vi "DLL-based calc.vi"() -> ()   [LabVIEW 2018]
uses:
  D:/Users_Data/Dmitriy_T/Documents/Tracker/TestVI's/Calculus2/Calculus.dll
  Calculus.dll
  <userlib>/_OpenG.lib/numeric/numeric.llb/Random Number Within Range - DBL__ogtk.vi
  <vilib>/Analysis/NI_AALBase.lvlib
panel:
  out "size(s)":i32
  out "Image Display":T1(plugin-control)
  in  "Y":i32=250
  in  "X":i32=300
  in  "Image":bool
  out "variance, us":dbl format="%0.2f"
  out "standard deviation, us":dbl format="%0.2f"
  out "mean per cycle, us":dbl format="%0.2f"
  in  "N tests":i32=10000
  out "Randoms":T2(graph)
  out "error out":errorcluster
  in  "Exit button":bool
  in  "Subtract":bool
  in  "Add":bool
  out "Result":i32
  in  "B":i32
  in  "A":i32
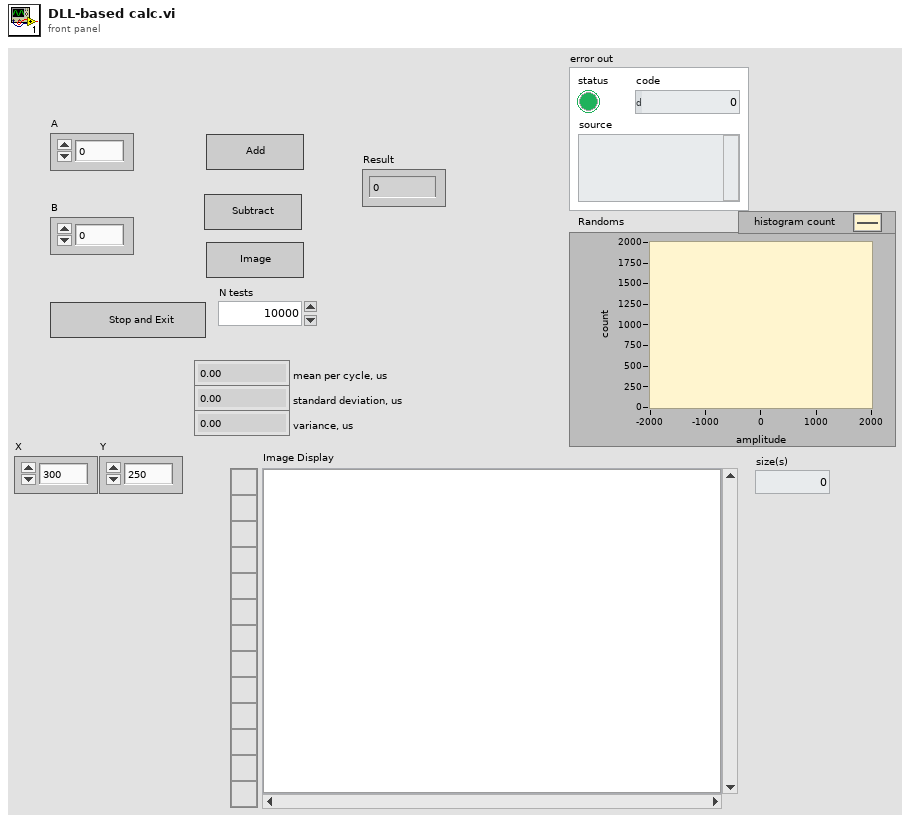
[diagram p1: front panel]
types:
  T1 = typedef "IMAQ Image.ctl" = refnum<image>
  T2 = cluster{"X Values":dbl[], "Histogram: h(x)":i32[]}
  T3 = typedef "Image Type" = u32
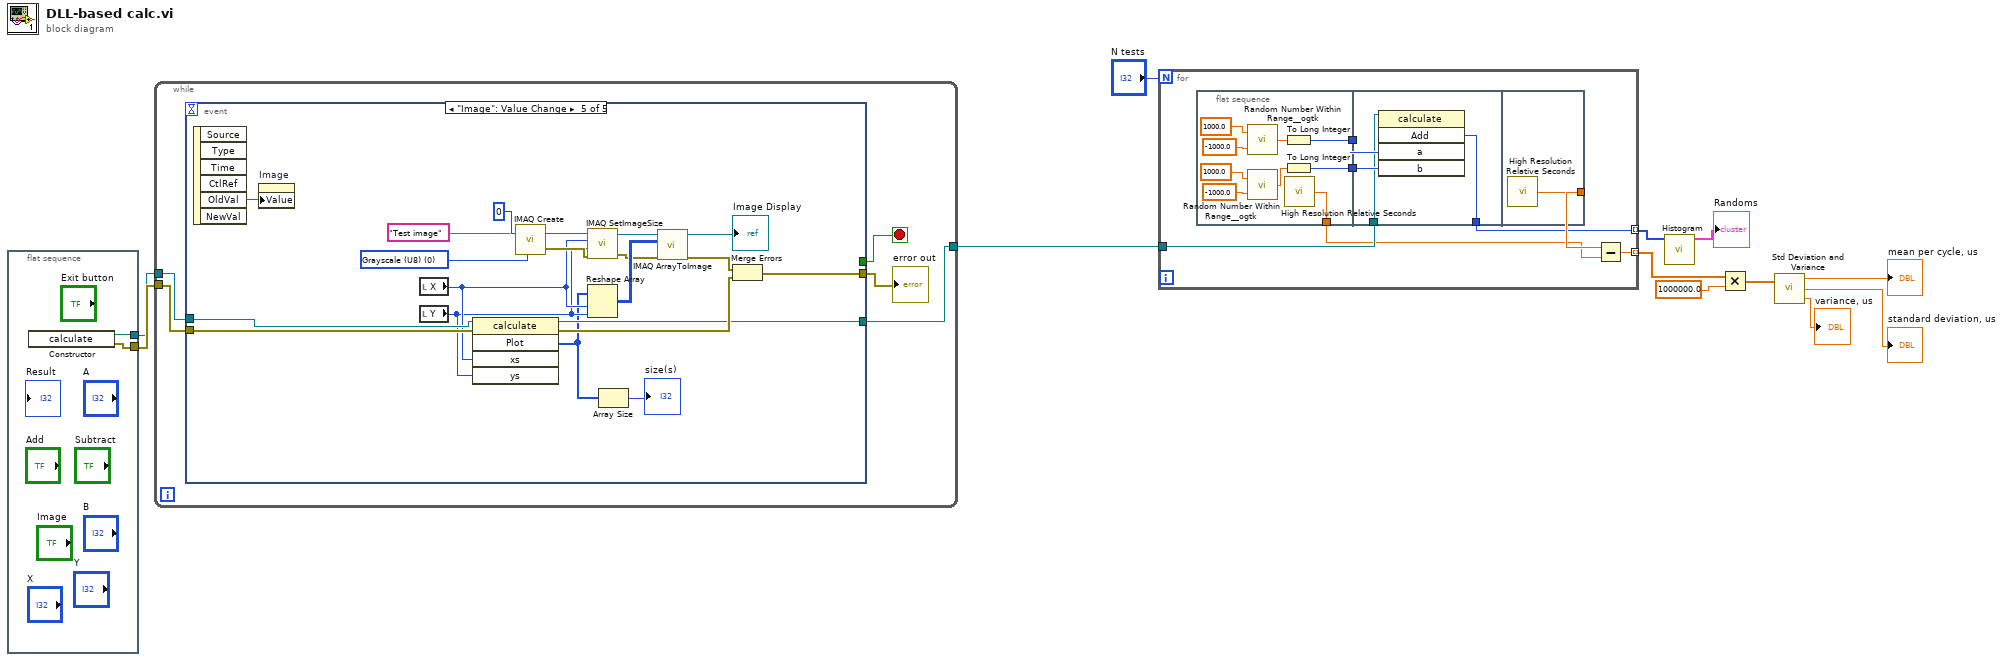
[diagram p0: block diagram]
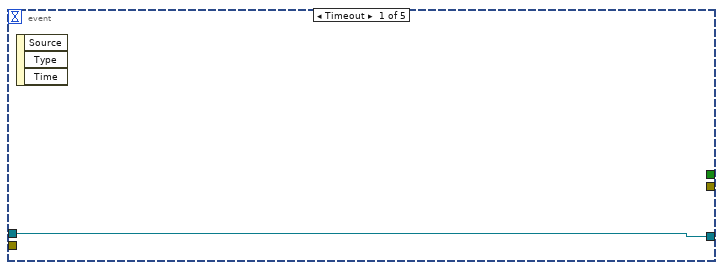
[diagram p2: hidden frame]
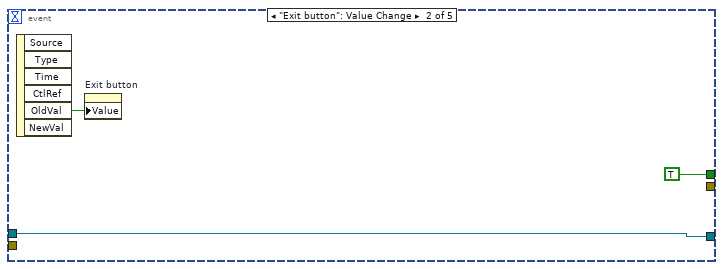
[diagram p3: hidden frame]
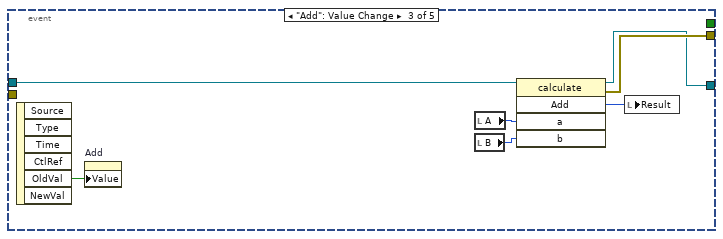
[diagram p4: hidden frame]
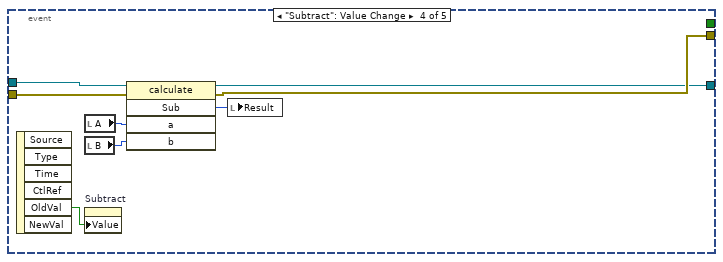
[diagram p5: hidden frame]
diagram:
  n1 = flat-sequence {
    tunnel: [w14] -> w11
    tunnel: [w13] -> w12
    frame #0 {
      n2 = constructor class="calculate"() -> (reference out=w14:refnum<k24>, error out=w13:errorcluster)  [unwired: 3 in, 1 out]
    }
  }
  n3 = while {
    tunnel: w11 -> [w18]
    tunnel: w12 -> [w17]
    tunnel: [w15] -> w10
    stop <- w19 stop-if-true
    n4 = event shown="[4] \"Image\": Value Change" {
      selector: _ -> [_ _ _ _ _]
      dyn-events: _ -> [_ _ _ _ _]
      timeout: _ -> [_ _ _ _ _]
      tunnel: [_ TRUE _ _ _] -> w19
      tunnel: w18 -> [w20 w21 w30 w38 w58]
      tunnel: w17 -> [_ _ _ w34 w57]
      tunnel: [_ _ w26 w33 w48] -> w16
      tunnel: [w20 w21 w24 w31 w54] -> w15
      event Timeout {
        n5 = event-data() -> ()  [unwired: 1 in, 3 out]
      }
      event "Exit button": Value Change {
        n6 = event-data() -> ("OldVal"=w22:bool)  [unwired: 1 in, 5 out]
        n7 = property on="Exit button" class="Bool (strict)"("Value"=w22) -> ()  [unwired: 2 in, 2 out]
      }
      event "Add": Value Change {
        n8 = event-data() -> ("OldVal"=w25:bool)  [unwired: 1 in, 5 out]
        n9 = property on="Add" class="Bool (strict)"("Value"=w25) -> ()  [unwired: 2 in, 2 out]
        n10 = local read "A"() -> (w29:i32)
        n11 = local read "B"() -> (w28:i32)
        n12 = invoke class="calculate" method="Add"(reference=w30, "a"=w29, "b"=w28) -> (reference out=w24:refnum<k24>, error out=w26:errorcluster, "Add"=w27:i32)  [unwired: 2 in, 2 out]
        n13 = local write "Result"(w27) -> ()
      }
      event "Subtract": Value Change {
        n14 = event-data() -> ("OldVal"=w32:bool)  [unwired: 1 in, 5 out]
        n15 = local read "A"() -> (w37:i32)
        n16 = local read "B"() -> (w36:i32)
        n17 = property on="Subtract" class="Bool (strict)"("Value"=w32) -> ()  [unwired: 2 in, 2 out]
        n18 = invoke class="calculate" method="Sub"(reference=w38, error in=w34, "a"=w37, "b"=w36) -> (reference out=w31:refnum<k24>, error out=w33:errorcluster, "Sub"=w35:i32)  [unwired: 1 in, 2 out]
        n19 = local write "Result"(w35) -> ()
      }
      event "Image": Value Change {
        w51 = T3 0 items=["Grayscale (U8)", "Grayscale (I16)", "Grayscale (SGL)", "Complex (CSG)", "RGB (U32)", "HSL (U32)", "RGB (U64)", "Grayscale (U16)"] ("Image Type")
        n20 = event-data() -> ("OldVal"=w55:bool)  [unwired: 1 in, 5 out]
        n21 = property on="Image" class="Bool (strict)"("Value"=w55) -> ()  [unwired: 2 in, 2 out]
        n22 = local read "X"() -> (w47:i32)
        n23 = local read "Y"() -> (w46:i32)
        n24 = invoke class="calculate" method="Plot"(reference=w58, error in=w57, "xs"=w47, "ys"=w46) -> (reference out=w54:refnum<k24>, error out=w56:errorcluster, "Plot"=w40:u8[])  [unwired: 1 in, 2 out]
        n25 = call "IMAQ Create"("Border Size"=0, "Image Name"="Test image", "Image Type"=w51) -> ("New Image"=w50:T1, "error out"=w49:errorcluster)  [unwired: 2 in]
        n26 = call "IMAQ SetImageSize"("error in (no error)"=w49, "Y Resolution"=w46, "X Resolution"=w47, "Image"=w50) -> ("error out"=w43:errorcluster, "Image Out"=w45:T1)  [unwired: 1 in]
        n27 = Reshape Array(w40, w47, w46) -> (w53:u8[][])
        n28 = Array Size(array=w40) -> (size(s)=→"size(s)":i32)
        n29 = call "IMAQ ArrayToImage"("error in (no error)"=w43, "Image Pixels (U8)"=w53, "Image"=w45) -> ("error out"=w42:errorcluster, "Image Out"=→"Image Display":T1)  [unwired: 7 in]
        n30 = Merge Errors(w42, w56) -> (w48:errorcluster)
      }
    }
    "error out" <- w16
  }
  n31 = for {
    N: "N tests" -> [_]
    tunnel: w10 -> [w63]
    tunnel: [w60] -> w8 mode=indexing
    tunnel: [w59] -> w6 mode=indexing
    n32 = flat-sequence {
      tunnel: [w69] -> w65
      tunnel: [w67] -> w64
      tunnel: [w66] -> w61
      tunnel: w65 -> [w78]
      tunnel: w64 -> [w77]
      tunnel: w63 -> [w76]
      tunnel: [w75] -> w60
      tunnel: [w79] -> w62
      frame #0 {
        n33 = call-poly <userlib>:"Random Number Within Range__ogtk.vi"("High"=1000.0, "Low"=-1000.0) -> ("Random Number"=w70:dbl)  [unwired: 3 in]
        n34 = call-poly <userlib>:"Random Number Within Range__ogtk.vi"("High"=1000.0, "Low"=-1000.0) -> ("Random Number"=w68:dbl)  [unwired: 3 in]
        n35 = To Long Integer(number=w70) -> (32bit integer=w69:i32)
        n36 = To Long Integer(number=w68) -> (32bit integer=w67:i32)
        n37 = call <vilib>:"High Resolution Relative Seconds.vi"() -> ("relative seconds"=w66:dbl)
      }
      frame #1 {
        n38 = invoke class="calculate" method="Add"(reference=w76, "a"=w78, "b"=w77) -> ("Add"=w75:i32)  [unwired: 2 in, 4 out]
      }
      frame #2 {
        n39 = call <vilib>:"High Resolution Relative Seconds.vi"() -> ("relative seconds"=w79:dbl)
      }
    }
    n40 = Subtract(x=w62, y=w61) -> (x-y=w59:dbl)
  }
  n41 = call <vilib>:"Histogram.vi"("X"=w8) -> ("Histogram Graph"=→"Randoms":T2)  [unwired: 7 in, 3 out]
  n42 = Multiply(x=w6, y=1000000.0) -> (x*y=w2:dbl[])
  n43 = call <vilib>:"Std Deviation and Variance.vi"("X"=w2) -> ("mean"=→"mean per cycle, us":dbl, "standard deviation"=→"standard deviation, us":dbl, "variance"=→"variance, us":dbl)  [unwired: 1 in]
